vi "Check Valid Message.vi"(8 "error in (no error)":errorcluster, 10 "Message":string, 11 "controller in":refnum<class "Generic Plugin.lvclass">) -> (0 "error out":errorcluster, 2 "Valid?":bool, 3 "controller out":refnum<class "Generic Plugin.lvclass">)   [LabVIEW 2020, in "Generic Plugin.lvclass"]
uses:
  Generic Plugin.lvclass
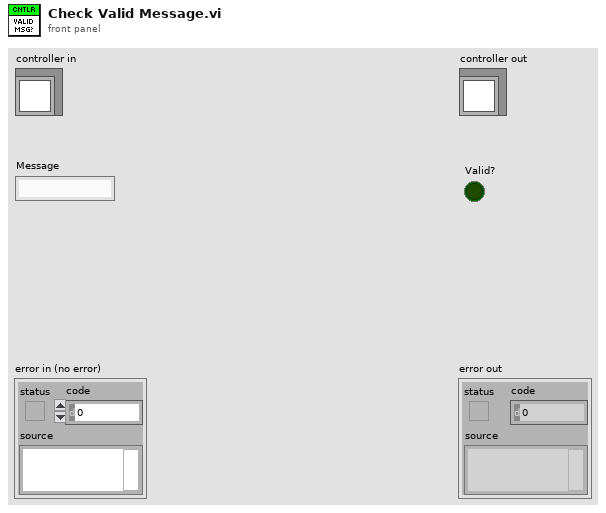
[diagram p1: front panel]
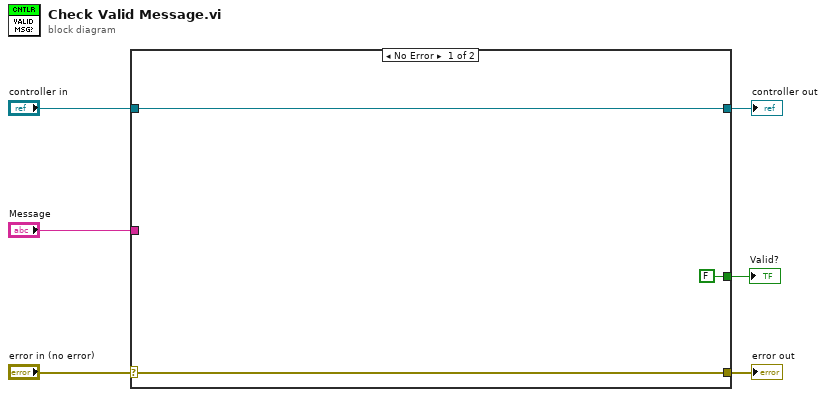
[diagram p0: block diagram]
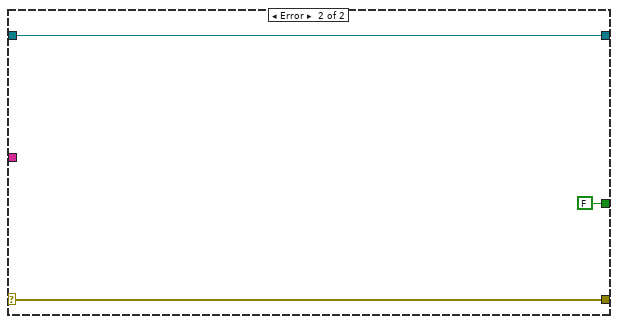
[diagram p2: hidden frame]
diagram:
  n1 = case shown="No Error" "error in (no error)" {
    selector: "error in (no error)" -> [w9 w12]
    tunnel: [w9 w12] -> w5
    tunnel: [w8 w11] -> w3
    tunnel: "controller in" -> [w8 w11]
    tunnel: "Message" -> [_ _]
    tunnel: [FALSE FALSE] -> w1
    frame No Error {
    }
    frame Error {
    }
  }
  "error out" <- w5
  "controller out" <- w3
  "Valid?" <- w1
